vi "Stop Acquisition.vi"(8 "error in (no error)":errorcluster, 11 "Hardware Resources in":T1) -> (0 "error out":errorcluster, 3 "Hardware Resources out":T1)   [LabVIEW 2026, in "Acquisition.lvlib"]
doc: "Stops the acquisition."
uses:
  Acquisition.lvlib
  Controls/Hardware Configuration.ctl
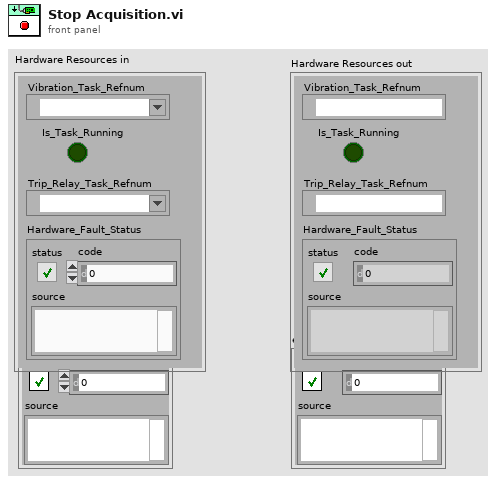
[diagram p1: front panel]
types:
  T1 = typedef "Acquisition.lvlib/Hardware Configuration.ctl" = cluster{"Vibration_Task_Refnum":refnum<k21>, "Is_Task_Running":bool, "Hardware_Fault_Status":errorcluster, "Trip_Relay_Task_Refnum":refnum<k21>}
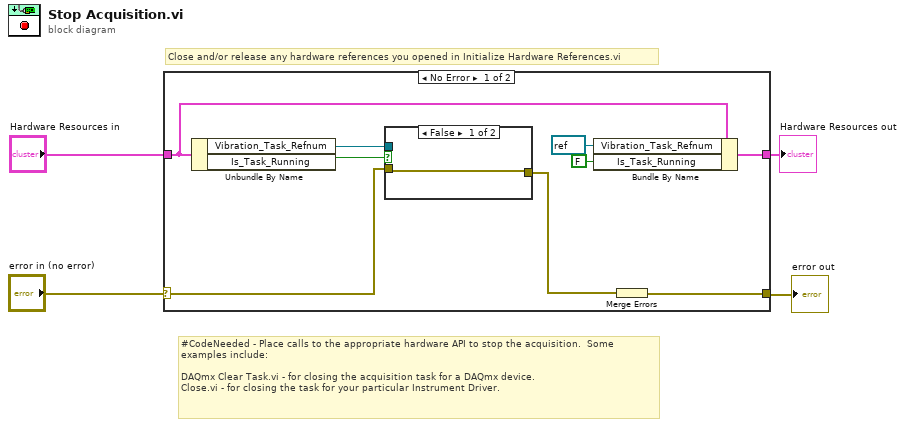
[diagram p0: block diagram]
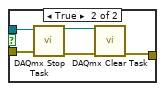
[diagram p2: hidden frame]
diagram:
  # "#CodeNeeded - Place calls to the appropriate hardware API to stop the acquisition.  Some examples include:\n\nDAQmx Clear Task.vi - for closing the acquisition task for a DAQmx device.\nClose.vi - for closing the task for your particular Instrument Driver."
  # "Close and/or release any hardware references you opened in Initialize Hardware References.vi"
  n1 = case shown="No Error" "error in (no error)" {
    selector: "error in (no error)" -> [w12 w21]
    tunnel: [w13 w21] -> w3
    tunnel: "Hardware Resources in" -> [w8 w20]
    tunnel: [w6 w20] -> w1
    frame No Error {
      n2 = Unbundle By Name(w8) -> ("Vibration_Task_Refnum"=w10:refnum<k21>, "Is_Task_Running"=w9:bool)
      n3 = case shown="False" w9 {
        tunnel: w12 -> [w14 w15]
        tunnel: [w14 w17] -> w11
        tunnel: w10 -> [_ w16]
        frame False {
        }
        frame True {
          n4 = call <vilib>:"DAQmx Stop Task.vi"("task/channels in"=w16, "error in"=w15) -> ("task out"=w19:refnum<k21>, "error out"=w18:errorcluster)  [unwired: 12 in]
          n5 = call <vilib>:"DAQmx Clear Task.vi"("task in"=w19, "error in"=w18) -> ("error out"=w17:errorcluster)  [unwired: 13 in]
        }
      }
      n6 = Bundle By Name(cluster=w8, "Vibration_Task_Refnum"=refnum<k21> refnum, "Is_Task_Running"=FALSE) -> (w6:T1)
      n7 = Merge Errors(w11) -> (w13:errorcluster)
    }
    frame Error {
    }
  }
  "error out" <- w3
  "Hardware Resources out" <- w1
